vi "rad_Configure Target Dialog.vi"(8 "Error In":errorcluster, 11 "Target Information in":T1={"Hostname"="", "Serial number"="", "Product name"="", "Product code"=0, "System status"="", "Credential type"=enum."None/Unlocked", "User added?"=FALSE, "Primary NIC"={"MAC address"="", "IP Address Request Mode"=2, "IP address"="", "Subnet mask"="", "Gateway"="", "DNS server"=""}} {"Primary NIC"."IP Address Request Mode" items=["Static"=1, "DHCP/Link-Local"=2, "Link-Local Only"=4, "DHCP Only"=8]}) -> (0 "Error Out":errorcluster, 3 "Target Information out":T1={"Hostname"="", "Serial number"="", "Product name"="", "Product code"=0, "System status"="", "Credential type"=enum."None/Unlocked", "User added?"=FALSE, "Primary NIC"={"MAC address"="", "IP Address Request Mode"=2, "IP address"="", "Subnet mask"="", "Gateway"="", "DNS server"=""}} {"Primary NIC"."IP Address Request Mode" items=["Static"=1, "DHCP/Link-Local"=2, "Link-Local Only"=4, "DHCP Only"=8]})   [LabVIEW 2020]
uses:
  TypeDefs/rad_Target Information.ctl
  TypeDefs/rad_Target Network Settings.ctl
panel:
  in  "IP Address Request Mode":i32(ring)=2 items=["Static"=1, "DHCP/Link-Local"=2, "Link-Local Only"=4, "DHCP Only"=8]
  in  "DNS":string
  in  "Gateway":string
  in  "Subnet Mask":string
  in  "IP Address":string
  in  "Host Name":string
  in  "Cancel":bool
  in  "OK":bool
  # "Network Configuration"
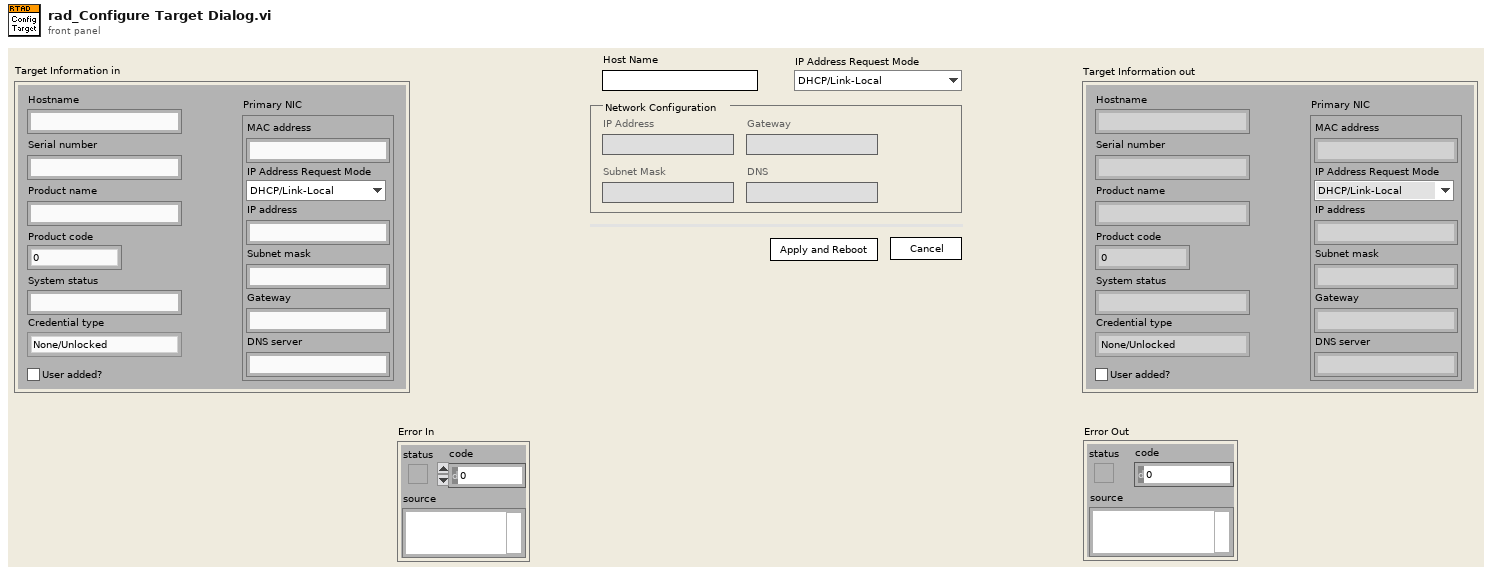
[diagram p1: front panel]
types:
  T1 = typedef "rad_Target Information.ctl" = cluster{"Hostname":string, "Serial number":string, "Product name":string, "Product code":i32, "System status":string, "Credential type":enum16{"None/Unlocked", "FTP Password", "NIAuth Credentials"}, "User added?":bool, "Primary NIC":T2}
  T2 = typedef "rad_Target Network Settings.ctl" = cluster{"MAC address":string, "IP Address Request Mode":i32, "IP address":string, "Subnet mask":string, "Gateway":string, "DNS server":string}
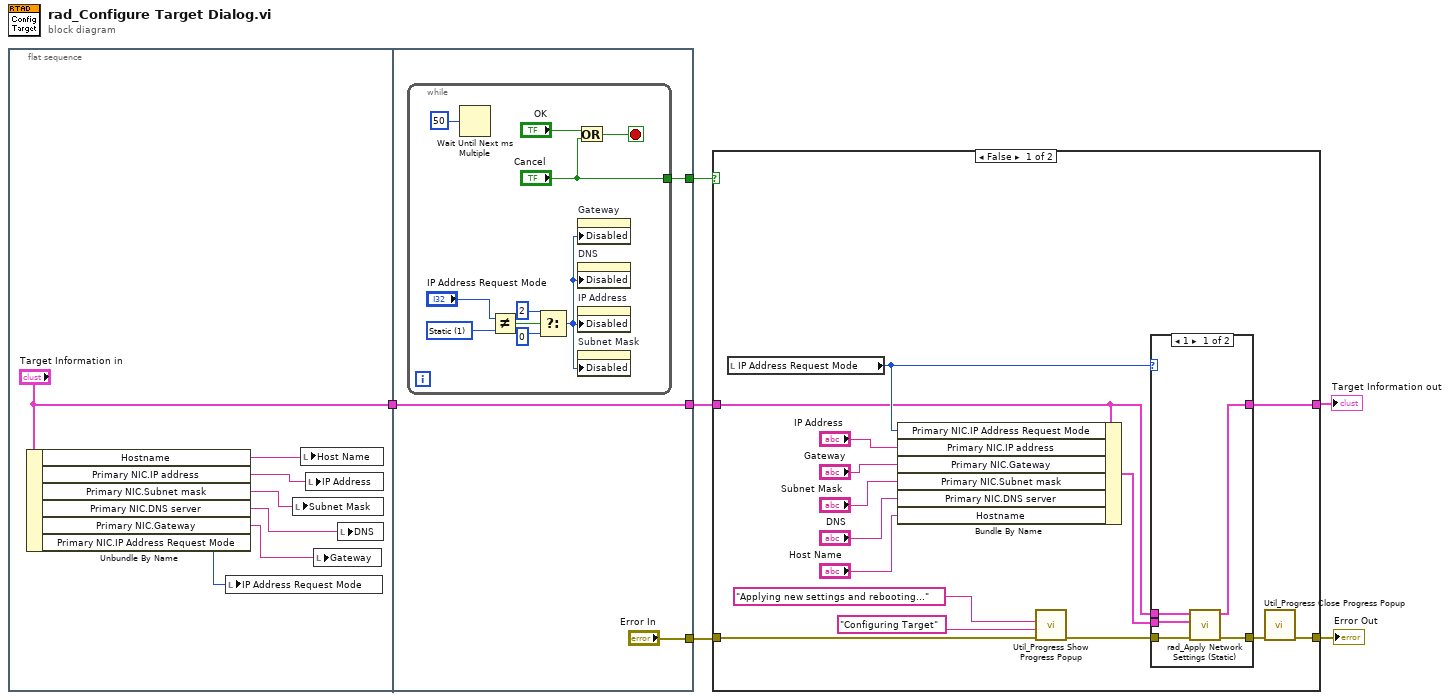
[diagram p0: block diagram]
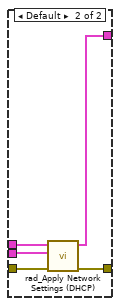
[diagram p2: hidden frame]
diagram:
  n1 = flat-sequence {
    tunnel: ["Target Information in"] -> w6
    tunnel: w6 -> [w15]
    tunnel: [w16] -> w3
    tunnel: [w15] -> w2
    tunnel: ["Error In"] -> w1
    frame #0 {
      n2 = Unbundle By Name("Target Information in") -> ("Hostname"=w13:string, "Primary NIC.IP address"=w12:string, "Primary NIC.Subnet mask"=w11:string, "Primary NIC.DNS server"=w10:string, "Primary NIC.Gateway"=w9:string, "Primary NIC.IP Address Request Mode"=w7:i32)
      n3 = local write "IP Address Request Mode"(w7) -> ()
      n4 = local write "Subnet Mask"(w11) -> ()
      n5 = local write "Host Name"(w13) -> ()
      n6 = local write "IP Address"(w12) -> ()
      n7 = local write "Gateway"(w9) -> ()
      n8 = local write "DNS"(w10) -> ()
    }
    frame #1 {
      n9 = while {
        tunnel: ["Cancel"] -> w16
        stop <- w24 stop-if-true
        w18 = 1 items=["Static"=1, "DHCP/Link-Local"=2, "Link-Local Only"=4, "DHCP Only"=8] ("IP Address Request Mode")
        n10 = Wait Until Next ms Multiple(millisecond multiple=u32 50) -> ()  [unwired: 1 out]
        n11 = Not Equal?(x="IP Address Request Mode", y=w18) -> (x != y?=w17:bool)
        n12 = Select(t=u8 2 ("Disabled"), s=w17, f=u8 0 ("Disabled")) -> (s? t:f=w20:u8)
        n13 = Or(x="OK", y="Cancel") -> (x .or. y?=w24:bool)
        n14 = property on="Gateway" class="Str"("Disabled"=w20) -> ()  [unwired: 2 in, 2 out]
        n15 = property on="DNS" class="Str"("Disabled"=w20) -> ()  [unwired: 2 in, 2 out]
        n16 = property on="IP Address" class="Str"("Disabled"=w20) -> ()  [unwired: 2 in, 2 out]
        n17 = property on="Subnet Mask" class="Str"("Disabled"=w20) -> ()  [unwired: 2 in, 2 out]
      }
    }
  }
  n18 = case shown="False" w3 {
    tunnel: w2 -> [w27 w53]
    tunnel: [w28 w53] -> w4
    tunnel: [w36 w52] -> w5
    tunnel: w1 -> [w39 w52]
    frame False {
      n19 = local read "IP Address Request Mode"() -> (w31:i32)
      n20 = Bundle By Name(cluster=w27, "Primary NIC.IP Address Request Mode"=w31, "Primary NIC.IP address"="IP Address", "Primary NIC.Gateway"="Gateway", "Primary NIC.Subnet mask"="Subnet Mask", "Primary NIC.DNS server"="DNS", "Hostname"="Host Name") -> (w30:T1)
      n21 = call "Util_Progress Show Progress Popup.vi"("error in (no error)"=w39, "Title"="Configuring Target", "Message"="Applying new settings and rebooting...") -> ("error out"=w37:errorcluster)  [unwired: 1 in, 7 out]
      n22 = case shown="1" w31 {
        tunnel: [w45 w50] -> w38
        tunnel: w37 -> [w46 w51]
        tunnel: w30 -> [w43 w48]
        tunnel: [w42 w49] -> w28
        tunnel: w27 -> [w44 w47]
        frame 1 {
          n23 = call "rad_Apply Network Settings (Static).vi"("error in (no error)"=w46, "Requested settings"=w43, "Existing settings"=w44) -> ("error out"=w45:errorcluster, "Target settings out"=w42:T1)  [unwired: 7 in]
        }
        frame Default {
          n24 = call "rad_Apply Network Settings (DHCP).vi"("error in (no error)"=w51, "Requested settings"=w48, "Existing settings"=w47) -> ("error out"=w50:errorcluster, "Target settings out"=w49:T1)  [unwired: 7 in]
        }
      }
      n25 = call "Util_Progress Close Progress Popup.vi"("error in (no error)"=w38) -> ("error out"=w36:errorcluster)  [unwired: 2 in, 8 out]
    }
    frame True {
    }
  }
  "Target Information out" <- w4
  "Error Out" <- w5
